vi "worker.vi"() -> ()   [LabVIEW 2014]
uses:
  <vilib>/addons/zeromq/socket_type.ctl
  <vilib>/addons/zeromq/zmq_context.lvclass
  <vilib>/addons/zeromq/zeromq.lvlib
  <vilib>/addons/zeromq/zmq_socket.lvclass
panel:
  out "String":string
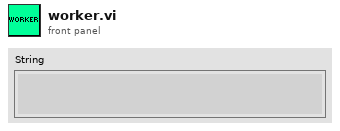
[diagram p1: front panel]
types:
  T1 = typedef "zeromq.lvlib/socket_type.ctl" = enum8{"ZMQ_PAIR", "ZMQ_PUB", "ZMQ_SUB", "ZMQ_REQ", "ZMQ_REP", "ZMQ_DEALER", "ZMQ_ROUTER", "ZMQ_PULL", "ZMQ_PUSH", "ZMQ_XPUB", "ZMQ_XSUB"}
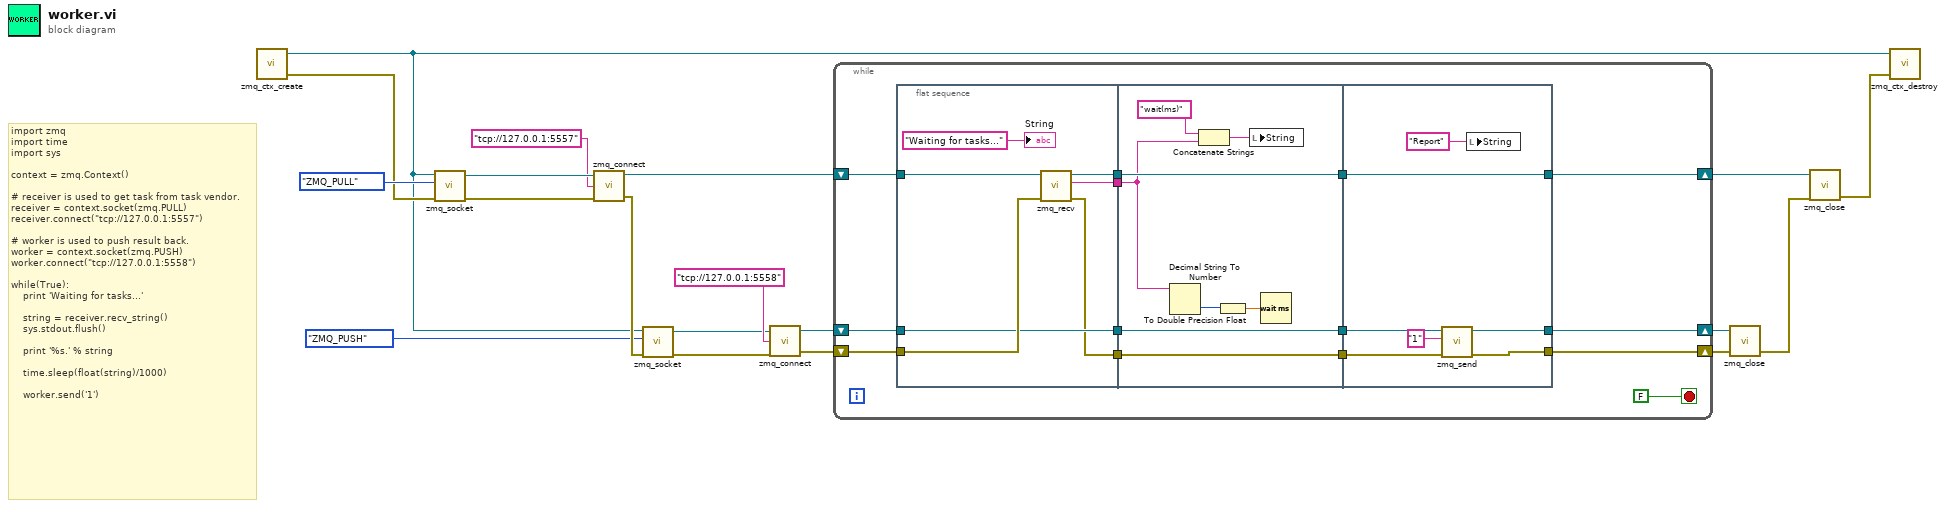
[diagram p0: block diagram]
diagram:
  # "import zmq\nimport time\nimport sys\n\ncontext = zmq.Context()\n\n# receiver is used to get task from task vendor.\nreceiver = context.socket(zmq.PULL)\nreceiver.connect(\"tcp://127.0.0.1:5557\")\n\n# worker is used to push result back.\nworker = context.socket(zmq.PUSH)\nworker.connect(\"tcp://127.0.0.1:5558\")\n\nwhile(True):\n    print 'Waiting for tasks...'\n\n    string = receiver.recv_string()\n    sys.stdout.flush()\n\n    print '%s.' % string\n\n    time.sleep(float(string)/1000)\n\n    worker.send('1')"
  n1 = call <vilib>:"zmq_ctx_create.vi"() -> ("error out"=w9:errorcluster, "context out"=w2:refnum<class "zmq_context.lvclass">)  [unwired: 4 in]
  n2 = call <vilib>:"zmq_socket.vi"("error in"=w9, "socket type"=socket_type."ZMQ_PULL", "context in"=w2) -> ("error out"=w17:errorcluster, "socket out"=w18:refnum<class "zmq_socket.lvclass">)  [unwired: 2 in, 1 out]
  n3 = call <vilib>:"zmq_connect.vi"("error in"=w17, "endpoint"="tcp://127.0.0.1:5557", "socket in"=w18) -> ("error out"=w6:errorcluster, "socket out"=w15:refnum<class "zmq_socket.lvclass">)  [unwired: 1 in]
  n4 = call <vilib>:"zmq_socket.vi"("error in"=w6, "socket type"=socket_type."ZMQ_PUSH", "context in"=w2) -> ("error out"=w11:errorcluster, "socket out"=w10:refnum<class "zmq_socket.lvclass">)  [unwired: 2 in, 1 out]
  n5 = call <vilib>:"zmq_connect.vi"("error in"=w11, "endpoint"="tcp://127.0.0.1:5558", "socket in"=w10) -> ("error out"=w8:errorcluster, "socket out"=w7:refnum<class "zmq_socket.lvclass">)  [unwired: 1 in]
  n6 = while {
    shift-right: [w30] -> w14
    shift-left: w15 -> [w32]
    shift-right: [w21] -> w4
    shift-left: w8 -> [w31]
    shift-right: [w20] -> w5
    shift-left: w7 -> [w24]
    stop <- FALSE stop-if-true
    n7 = flat-sequence {
      tunnel: w32 -> [w39]
      tunnel: w31 -> [w38]
      tunnel: [w40] -> w29
      tunnel: [w37] -> w28
      tunnel: [w35] -> w25
      tunnel: w24 -> [w35]
      tunnel: [w34] -> w22
      tunnel: w29 -> [w45]
      tunnel: w28 -> [w48]
      tunnel: [w48] -> w27
      tunnel: [w42] -> w26
      tunnel: w25 -> [w42]
      tunnel: [w41] -> w23
      tunnel: w22 -> [w41]
      tunnel: [w55] -> w30
      tunnel: w27 -> [w55]
      tunnel: w26 -> [w54]
      tunnel: w23 -> [w53]
      tunnel: [w52] -> w21
      tunnel: [w50] -> w20
      frame #0 {
        n8 = call <vilib>:"zmq_recv.vi"("error in"=w38, "socket in"=w39) -> ("error out"=w34:errorcluster, "data"=w40:string, "socket out"=w37:refnum<class "zmq_socket.lvclass">)  [unwired: 3 in, 2 out]
        "String" <- "Waiting for tasks..." ("String")
      }
      frame #1 {
        n9 = Decimal String To Number(string=w45) -> (number=w46:i32)  [unwired: 2 in, 1 out]
        n10 = Concatenate Strings("wait(ms)" ("string"), w45) -> (w44:string)
        n11 = To Double Precision Float(number=w46) -> (double precision float=w47:dbl)
        n12 = local write "String"(w44) -> ()
        n13 = Wait (ms)(milliseconds to wait=w47) -> ()  [unwired: 1 out]
      }
      frame #2 {
        n14 = call <vilib>:"zmq_send.vi"("error in"=w53, "data"="1", "socket in"=w54) -> ("error out"=w52:errorcluster, "socket out"=w50:refnum<class "zmq_socket.lvclass">)  [unwired: 4 in]
        n15 = local write "String"("Report" ("String")) -> ()
      }
    }
  }
  n16 = call <vilib>:"zmq_close.vi"("error in"=w4, "socket"=w5) -> ("error out"=w3:errorcluster)  [unwired: 3 in]
  n17 = call <vilib>:"zmq_close.vi"("error in"=w3, "socket"=w14) -> ("error out"=w13:errorcluster)  [unwired: 3 in]
  n18 = call <vilib>:"zmq_ctx_destroy.vi"("error in"=w13, "context in"=w2) -> ()  [unwired: 3 in, 1 out]
